vi "KH_DAQ_TURCK_FGlob_DAQmxDO.vi"(5 "Function (Recall One)":T1=enum."Recall one", 6 "Alarm":bool, 7 "PXI DO_Item":i32, 8 "err in":errorcluster caption="error", 9 "DXP Reset IN":bool[](array[boolean]), 10 "DXP Values IN":bool[](array[boolean]), 11 "DXP Value IN":bool) -> (0 "err out":errorcluster caption="error", 1 "DXP Reset OUT":bool[](array[boolean]), 2 "DXP Values OUT":bool[](array[boolean]), 3 "DXP Value OUT":bool)   [LabVIEW 2021]
uses:
  KH Turck EthernetIP 17.12/KH TURCK TypeDefs FGlob.ctl
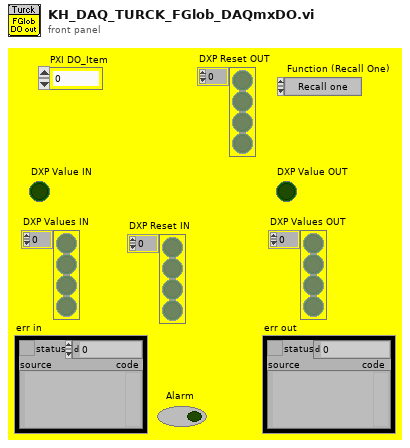
[diagram p1: front panel]
types:
  T1 = typedef "KH TURCK TypeDefs FGlob.ctl" = enum16{"Put one", "Put all", "Recall one", "Recall all"}
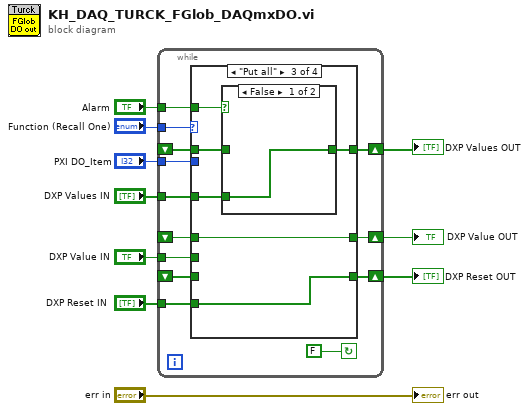
[diagram p0: block diagram]
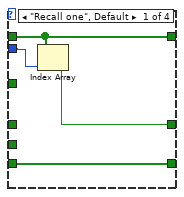
[diagram p2: hidden frame]
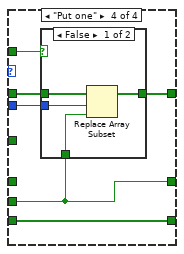
[diagram p5: hidden frame]
diagram:
  n1 = while {
    shift-right: [w21] -> w8
    shift-left: _ -> [w20]
    tunnel: "Function (Recall One)" -> [w22]
    tunnel: "PXI DO_Item" -> [w18]
    tunnel: "DXP Values IN" -> [w17]
    shift-right: [w19] -> w7
    shift-left: _ -> [w16]
    tunnel: "DXP Value IN" -> [w15]
    tunnel: "Alarm" -> [w14]
    tunnel: "DXP Reset IN" -> [w13]
    shift-right: [w12] -> w1
    shift-left: _ -> [w11]
    stop <- FALSE continue-if-true
    n2 = case shown="\"Put all\"" w22 {
      tunnel: [w27 w30 w33 w43] -> w21
      tunnel: w20 -> [w27 w30 w34 w44]
      tunnel: w18 -> [w26 _ _ w42]
      tunnel: [w25 w29 w36 w41] -> w19
      tunnel: w17 -> [_ _ w32 _]
      tunnel: w16 -> [_ w29 w36 _]
      tunnel: w15 -> [_ _ _ w41]
      tunnel: w14 -> [_ _ w35 w40]
      tunnel: w13 -> [_ _ w31 _]
      tunnel: [w24 w28 w31 w39] -> w12
      tunnel: w11 -> [w24 w28 _ w39]
      frame "Recall one", Default {
        n3 = Index Array(array=w27, index=w26) -> (element=w25:bool)
      }
      frame "Recall all" {
      }
      frame "Put all" {
        n4 = case shown="False" w35 {
          tunnel: [w37 w38] -> w33
          tunnel: w34 -> [_ w38]
          tunnel: w32 -> [w37 _]
          frame False {
          }
          frame True {
          }
        }
      }
      frame "Put one" {
        n5 = case shown="False" w40 {
          tunnel: w44 -> [w48 w49]
          tunnel: [w47 w49] -> w43
          tunnel: w42 -> [w46 _]
          tunnel: w41 -> [w45 _]
          frame False {
            n6 = Replace Array Subset(array=w48, new element=w45, index=w46) -> (w47:bool[])
          }
          frame True {
          }
        }
      }
    }
  }
  "DXP Values OUT" <- w8
  "DXP Value OUT" <- w7
  "DXP Reset OUT" <- w1
  "err out" <- "err in"
